vi "Sets the Beeper Mode.vi"(5 "Enable to Query":bool=TRUE, 7 "Enable to Sets":bool=TRUE, 8 "error in":errorcluster, 10 "Beeper Mode":u16(ring) items=["No Beep", "Beep on Pass", "Beep on Fail"], 11 "VISA resource name":refnum<visa-resource-name>) -> (0 "error out":errorcluster, 2 "Return the Beeper Mode":string, 3 "VISA resource name out":refnum<visa-resource-name>)   [LabVIEW 2011, in "DMM4.lvlib"]
uses:
  <instrlib>/DMM4/DMM4.lvlib
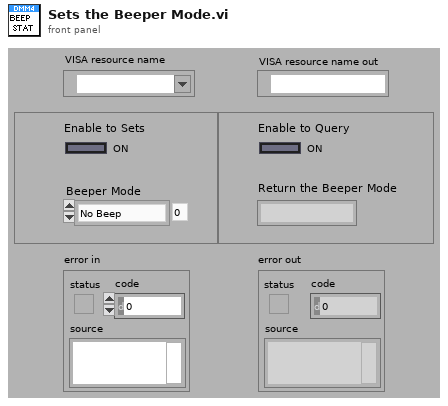
[diagram p1: front panel]
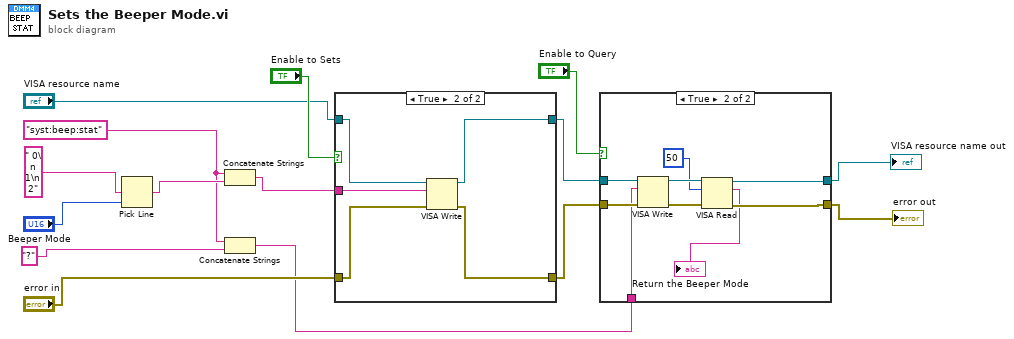
[diagram p0: block diagram]
diagram:
  w12 = "syst:beep:stat"
  n1 = Pick Line(multi-line string=" 0\n 1\n 2", line index="Beeper Mode") -> (output string=w13:string)  [unwired: 1 in]
  n2 = Concatenate Strings(w12, w13) -> (w7:string)
  n3 = Concatenate Strings(w12, "?") -> (w3:string)
  n4 = case shown="True" "Enable to Sets" {
    tunnel: "VISA resource name" -> [w17 w22]
    tunnel: "error in" -> [w16 w21]
    tunnel: [w17 w20] -> w5
    tunnel: [w16 w19] -> w4
    tunnel: w7 -> [_ w18]
    frame False {
    }
    frame True {
      n5 = VISA Write(VISA resource name=w22, write buffer=w18, error in (no error)=w21) -> (VISA resource name out=w20:refnum<visa-resource-name>, error out=w19:errorcluster)  [unwired: 1 out]
    }
  }
  n6 = case shown="True" "Enable to Query" {
    tunnel: w5 -> [w24 w33]
    tunnel: w4 -> [w23 w32]
    tunnel: w3 -> [_ w31]
    tunnel: [w24 w28] -> w2
    tunnel: [w23 w27] -> w1
    frame False {
    }
    frame True {
      n7 = VISA Write(VISA resource name=w33, write buffer=w31, error in (no error)=w32) -> (VISA resource name out=w30:refnum<visa-resource-name>, error out=w29:errorcluster)  [unwired: 1 out]
      n8 = VISA Read(VISA resource name=w30, byte count=u32 50, error in (no error)=w29) -> (VISA resource name out=w28:refnum<visa-resource-name>, read buffer=→"Return the Beeper Mode":string, error out=w27:errorcluster)  [unwired: 1 out]
    }
  }
  "VISA resource name out" <- w2
  "error out" <- w1
